vi "Class Tree_Arrow Control.vi"(7 "Direction":enum16{"Down", "Up"}(ring), 8 "error in (no error)":errorcluster, 11 "Tree ref":refnum<vi>) -> (0 "error out":errorcluster, 2 "discard":bool)   [LabVIEW 2023]
doc: "On kep up or down, go to next displayed item in list. Assume that keyboard navigation is in use, and replace the last selected item. THis will probably fila is multiple items are already selected, and so should be disabled if that's the case."
panel:
  out "first item":bool
  out "last item":bool
  in  "Tree":string[](tree)
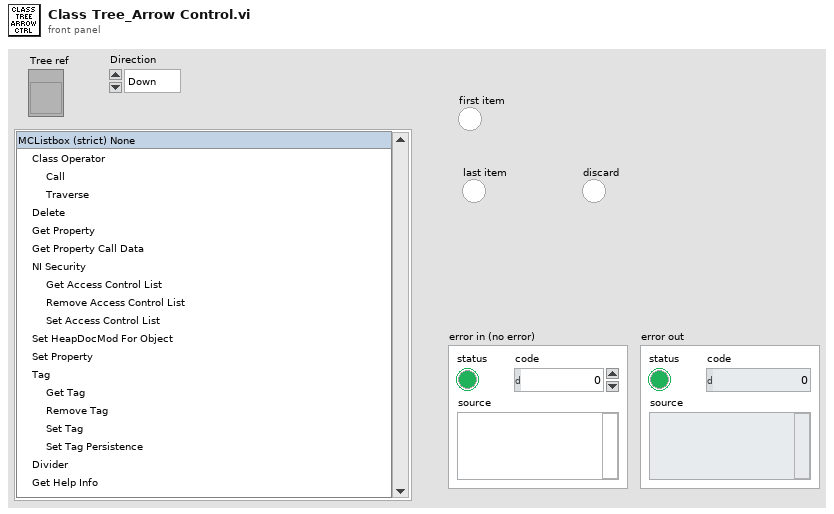
[diagram p1: front panel]
types:
  T1 = typedef "Type Descriptor Enumeration__ogtk.ctl" = enum8{"<Null>", "I8", "I16", "I32", "I64", "U8", "U16", "U32", "U64", "SGL", "DBL", "EXT", "CSG", "CDB", "CXT", "0x0F", "0x10", "0x11", "0x12", "0x13", "0x14", "Enum U8", "Enum U16", "Enum U32", "Enum U64", "SGL PQ", "DBL PQ", "EXT PQ", "CSG PQ", "CDB PQ", "CXT PQ", "0x1F", "0x20", "Boolean", "0x22", "0x23", "0x24", "0x25", "0x26", "0x27", "0x28", "0x29", "0x2A", "0x2B", "0x2C", "0x2D", "0x2E", "0x2F", "String", "0x31", "Path", "Pict", "0x34", "0x35", "0x36", "DAQ", "0x38", "0x39", "0x3A", "0x3B", "0x3C", "0x3D", "0x3E", "0x3F", "Array", "0x41", "0x42", "0x43", "0x44", "0x45", "0x46", "0x47", "0x48", "0x49", "0x4A", "0x4B", "0x4C", "0x4D", "0x4E", "0x4F", "Cluster", "0x51", "0x52", "Variant", "Waveform", "0x55", "0x56", "0x57", "0x58", "0x59", "0x5A", "0x5B", "0x5C", "0x5D", "0x5E", "Fixed Point", "0x60", "0x61", "0x62", "0x63", "0x64", "0x65", "0x66", "0x67", "0x68", "0x69", "0x6A", "0x6B", "0x6C", "0x6D", "0x6E", "0x6F", "Refnum", "0x71", "0x72", "Set Collection", "Map Collection"}
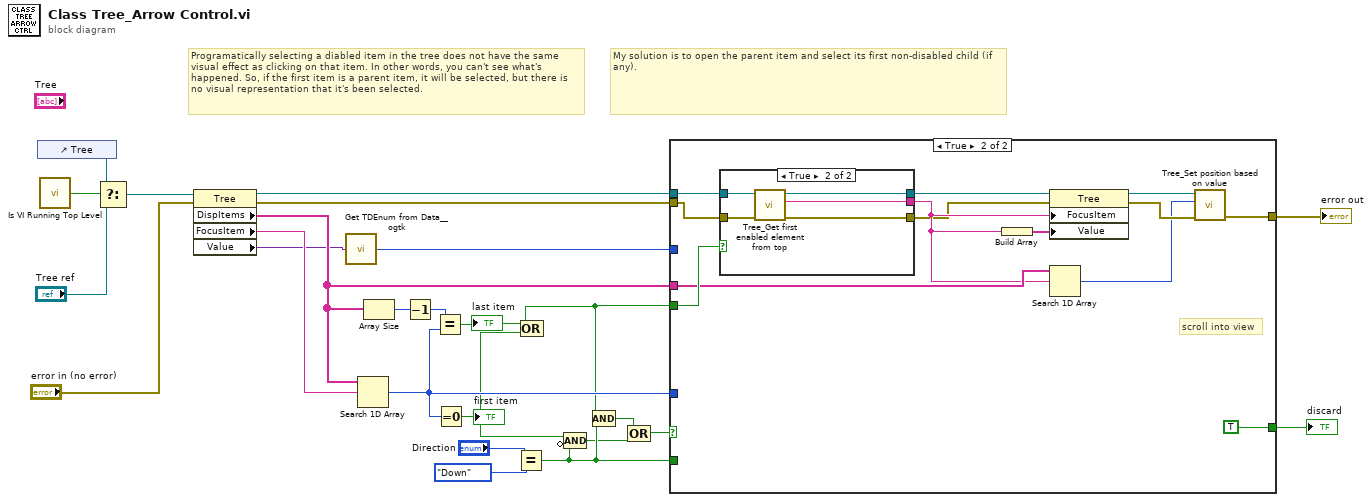
[diagram p0: block diagram]
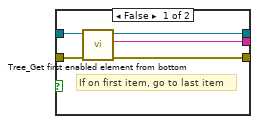
[diagram p3: hidden frame]
diagram:
  # "My solution is to open the parent item and select its first non-disabled child (if any)."
  # "Programatically selecting a diabled item in the tree does not have the same visual effect as clicking on that item. In other words, you can't see what's happened. So, if the first item is a parent item, it will be selected, but there is no visual representation that it's been selected."
  n1 = control-ref of="Tree"() -> (w24:refnum<vi>)
  n2 = call "Is VI Running Top Level.vi"() -> ("Top Level?"=w19:bool)  [unwired: 5 in]
  n3 = Select(t=w24, s=w19, f="Tree ref") -> (s? t:f=w20:refnum<vi>)
  n4 = property class="Tree"(reference=w20, error in="error in (no error)") -> (reference out=w7:refnum<vi>, error out=w5:errorcluster, "DispItems"=w8:string[], "FocusItem"=w21:string, "Value"=w2:variant)
  n5 = call <userlib>:"Get TDEnum from Data__ogtk.vi"("Data"=w2) -> ("Type Descriptor Enumeration"=w1:T1)  [unwired: 4 in]
  n6 = Search 1D Array(1D array=w8, element=w21) -> (index of element=w15:i32)  [unwired: 1 in]
  n7 = Array Size(array=w8) -> (size(s)=w17:i32)
  n8 = Decrement(x=w17) -> (x-1=w16:i32)
  n9 = Equal?(x=w16, y=w15) -> (x = y?=w14:bool)
  "last item" <- w14
  n10 = Equal To 0?(x=w15) -> (x = 0?=w13:bool)
  "first item" <- w13
  n11 = Equal?(x="Direction", y=enum16{"Down", "Up"}."Down" ("Direction")) -> (x = y?=w12:bool)
  n12 = Compound Arithmetic op=OR(w14, w13) -> ()  [unwired: 1 out]
  n13 = Compound Arithmetic op=AND(w13, invert w12) -> (w10:bool)
  n14 = Compound Arithmetic op=AND(w14, w12) -> (w11:bool)
  n15 = Compound Arithmetic op=OR(w11, w10) -> (w9:bool)
  n16 = case shown="True" w9 {
    tunnel: w8 -> [_ w37]
    tunnel: w15 -> [_ _]
    tunnel: w12 -> [_ _]
    tunnel: w14 -> [_ w38]
    tunnel: w7 -> [_ w26]
    tunnel: [w25 w33] -> w6
    tunnel: w5 -> [w25 w28]
    tunnel: [_ TRUE ("discard")] -> w3
    tunnel: w1 -> [_ _]
    frame False {
    }
    frame True {
      # "scroll into view"
      n17 = case shown="True" w38 {
        tunnel: [w39 w45] -> w31
        tunnel: w26 -> [w41 w48]
        tunnel: w28 -> [w43 w47]
        tunnel: [w42 w46] -> w29
        tunnel: [w40 w44] -> w27
        frame False {
          # "If on first item, go to last item"
          n18 = call "Tree_Get first enabled element from bottom.vi"("error in (no error)"=w43, "TreeControl Ref"=w41) -> ("error out"=w42:errorcluster, "First Element Tag"=w39:string, "Tree Control Ref Out"=w40:refnum<vi>)  [unwired: 7 in]
        }
        frame True {
          n19 = call "Tree_Get first enabled element from top.vi"("error in (no error)"=w47, "Tree Control Ref"=w48) -> ("error out"=w46:errorcluster, "First Enabled Element"=w45:string, "Tree Control Ref Out"=w44:refnum<vi>)  [unwired: 7 in]
        }
      }
      n20 = Build Array(w31) -> (w30:string[])
      n21 = property class="Tree"(reference=w27, error in=w29, "FocusItem"=w31, "Value"=w30) -> (reference out=w34:refnum<vi>, error out=w36:errorcluster)
      n22 = Search 1D Array(1D array=w37, element=w31) -> (index of element=w35:i32)  [unwired: 1 in]
      n23 = call "Tree_Set position based on value.vi"("error in (no error)"=w36, "Selected Row"=w35, "Tree Ref"=w34) -> ("error out"=w33:errorcluster)  [unwired: 7 in, 1 out]
    }
  }
  "error out" <- w6
  "discard" <- w3
